vi "Write Array to 3.vi"(11 "Test Case In":refnum<class "Tests Event MessengerM.lvclass">) -> (0 "error out":errorcluster, 3 "Test Case Out":refnum<class "Tests Event MessengerM.lvclass">)   [LabVIEW 2020, in "Tests Event MessengerM.lvclass"]
uses:
  Tests Event MessengerM.lvclass
  Tests Event MessengerM.lvclass/Tests Event MessengerM.ctl
  <vilib>/Astemes/LUnit/Test Case.lvclass
  <vilib>/Analysis/NI_AALBase.lvlib
  <vilib>/Analysis/1siggen.llb/Ramp Pattern by Samples.vi
  35e05ace-a30a-48ea-a6e4-616ba598f661.vi
  711b8d36-41a8-4866-9f20-9f97b272b204.vi
  ef278ddd-1243-4bda-a5f7-6430f324e75b.vi
  ddb176f8-0384-49d9-9061-ef500680968d.vi
  5b44630a-5ea4-46ee-9356-0a1333bf0eb8.vi
  42043d21-fccf-444c-821b-517e42210671.vi
panel:
  out "x = y? 2":bool
  out "x = y? 1":bool
  out "x = y? 0":bool
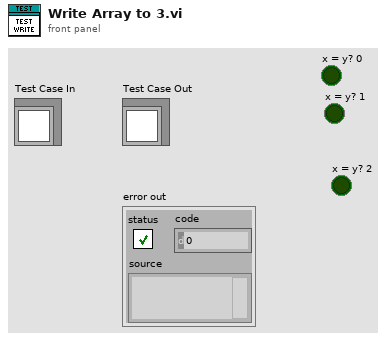
[diagram p1: front panel]
types:
  T1 = typedef "Event MessengerM-a[.](dbl).lvlib/))Channel.ctl" = refnum<queue>
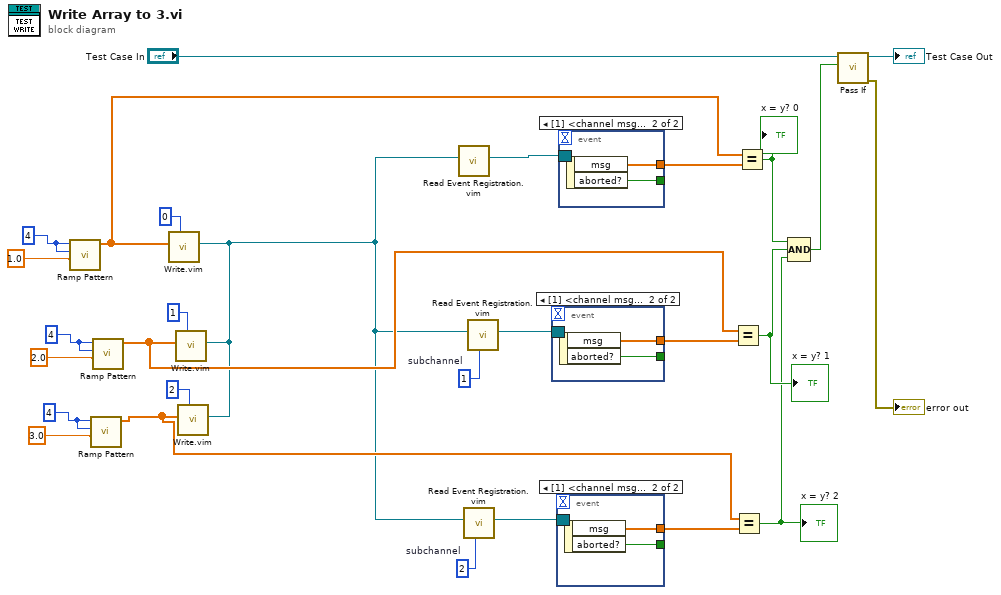
[diagram p0: block diagram]
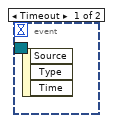
[diagram p2: hidden frame]
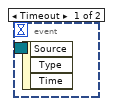
[diagram p3: hidden frame]
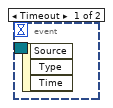
[diagram p4: hidden frame]
diagram:
  w5 = 4 ("samples")
  w6 = 4 ("samples")
  w11 = 4 ("samples")
  w1 = 2  # subchannel
  w2 = 1  # subchannel
  n1 = call-poly <vilib>:"Ramp Pattern.vi"("start"=1.0, "end"=w11, "samples"=w11) -> ("Ramp Pattern"=w19:dbl[])  [unwired: 7 in, 1 out]
  n2 = call-poly <vilib>:"Ramp Pattern.vi"("start"=3.0, "end"=w5, "samples"=w5) -> ("Ramp Pattern"=w16:dbl[])  [unwired: 7 in, 1 out]
  n3 = call-poly <vilib>:"Ramp Pattern.vi"("start"=2.0, "end"=w6, "samples"=w6) -> ("Ramp Pattern"=w18:dbl[])  [unwired: 7 in, 1 out]
  n4 = call "Write.vim"("subchannel"=0 ("subchannel (0)"), "element"=w19) -> ("channel"=w15:T1)  [unwired: 8 in, 1 out]
  n5 = call "Write.vim"("channel"=w15, "subchannel"=1 ("subchannel (0)"), "element"=w18) -> ()  [unwired: 8 in, 1 out]
  n6 = call "Write.vim"("channel"=w15, "subchannel"=2 ("subchannel (0)"), "element"=w16) -> ()  [unwired: 8 in, 1 out]
  n7 = call "Read Event Registration.vim"("channel"=w15) -> ("event registration refnum"=w22:refnum<event-registration>)  [unwired: 10 in]
  n8 = call "Read Event Registration.vim"("subchannel"=w1, "channel"=w15) -> ("event registration refnum"=w20:refnum<event-registration>)  [unwired: 9 in]
  n9 = call "Read Event Registration.vim"("subchannel"=w2, "channel"=w15) -> ("event registration refnum"=w21:refnum<event-registration>)  [unwired: 9 in]
  n10 = event shown="[1] <channel msg>: User Event" {
    selector: w21 -> [_ _]
    dyn-events: _ -> [_ _]
    timeout: _ -> [_ _]
    tunnel: [_ w30] -> w17
    tunnel: [_ w29] -> _
    event Timeout {
      n11 = event-data() -> ()  [unwired: 1 in, 3 out]
    }
    event User Event {
      n12 = event-data() -> ("msg"=w30:dbl[], "aborted?"=w29:bool)  [unwired: 1 in]
    }
  }
  n13 = event shown="[1] <channel msg>: User Event" {
    selector: w20 -> [_ _]
    dyn-events: _ -> [_ _]
    timeout: _ -> [_ _]
    tunnel: [_ w32] -> w23
    tunnel: [_ w31] -> _
    event Timeout {
      n14 = event-data() -> ()  [unwired: 1 in, 3 out]
    }
    event User Event {
      n15 = event-data() -> ("msg"=w32:dbl[], "aborted?"=w31:bool)  [unwired: 1 in]
    }
  }
  n16 = event shown="[1] <channel msg>: User Event" {
    selector: w22 -> [_ _]
    dyn-events: _ -> [_ _]
    timeout: _ -> [_ _]
    tunnel: [_ w34] -> w25
    tunnel: [_ w33] -> _
    event Timeout {
      n17 = event-data() -> ()  [unwired: 1 in, 3 out]
    }
    event User Event {
      n18 = event-data() -> ("msg"=w34:dbl[], "aborted?"=w33:bool)  [unwired: 1 in]
    }
  }
  n19 = Equal?(x=w18, y=w17) -> (x = y?=w13:bool)
  "x = y? 1" <- w13
  n20 = Equal?(x=w16, y=w23) -> (x = y?=w12:bool)
  "x = y? 2" <- w12
  n21 = Equal?(x=w19, y=w25) -> (x = y?=w14:bool)
  "x = y? 0" <- w14
  n22 = Compound Arithmetic op=AND(w14, w13, w12) -> (w24:bool)
  n23 = call <vilib>:"Pass If.vi"("Pass?"=w24, "LUnit Test Case In"="Test Case In") -> ("error out"=→"error out":errorcluster, "LUnit Test Case Out"=→"Test Case Out":refnum<class "Tests Event MessengerM.lvclass">)  [unwired: 8 in]
